vi "Handle Chart Settings.vi"(6 "Table Setting Name in":string, 7 "Write Ctl? (F:Read)":bool, 8 "error in (no error)":errorcluster, 9 "Table Ref":refnum<vi>, 11 "Save Restore Settings in":refnum<class "Save Restore Settings.lvclass">) -> (0 "error out":errorcluster, 1 "Sub Controls":T1[](array[typedef]), 3 "Save Restore Settings out":refnum<class "Save Restore Settings.lvclass">)   [LabVIEW 2016, in "Save Restore Settings.lvclass"]
uses:
  <userlib>/_MGI/Application Control/MGI Save Restore Settings/Save Restore Settings.lvclass
  <userlib>/_MGI/Application Control/MGI Save Restore Settings/Control Info.ctl
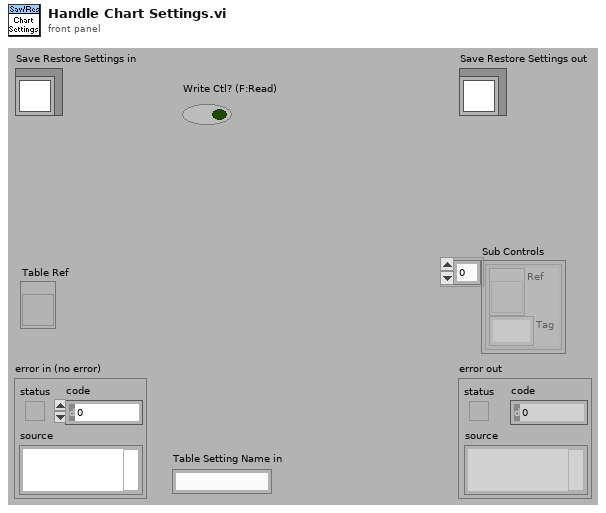
[diagram p1: front panel]
types:
  T1 = typedef "Save Restore Settings.lvclass/Control Info.ctl" = cluster{"Ref":refnum<vi>, "Tag":string}
  T2 = cluster{"XScaleIdx":u32, "YScaleIdx":u32, "Info":cluster{"Plot Color":u32, "Plot Interpolation":u8, "Point Style":u8, "Line Style":u8, "Fill/Pt. Color":u32, "Line Width":u8, "Bar Plot Style":u8, "Fill To":i16}}
  T3 = cluster{"Plot Color":u32, "Plot Interpolation":u8, "Point Style":u8, "Line Style":u8, "Fill/Pt. Color":u32, "Line Width":u8, "Bar Plot Style":u8, "Fill To":i16}
  T4 = cluster{"XScaleIdx":u32, "YScaleIdx":u32, "Info":cluster{"Plot Color":u32, "Plot Interpolation":u8, "Point Style":u8, "Line Style":u8, "Fill/Pt. Color":u32, "Line Width":u8, "Bar Plot Style":u8, "Fill To":i16}}[]
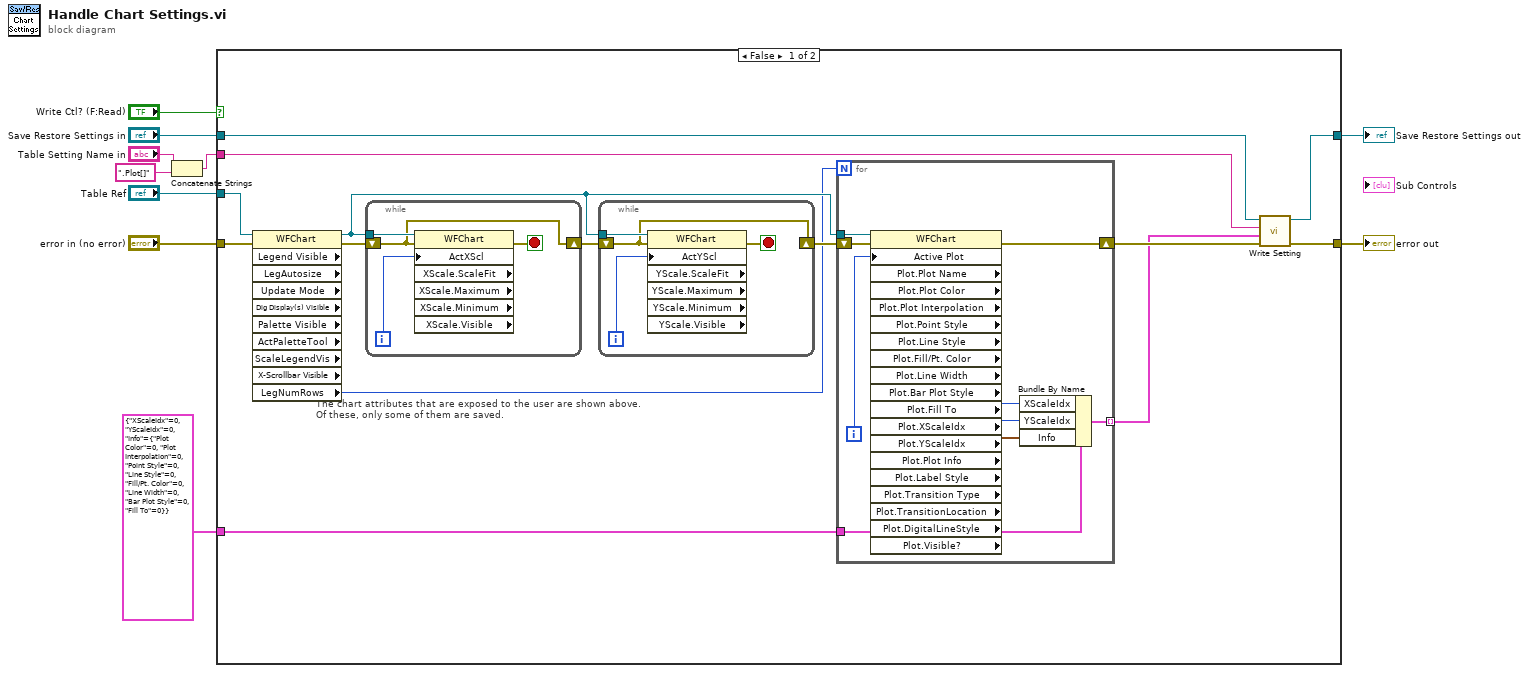
[diagram p0: block diagram]
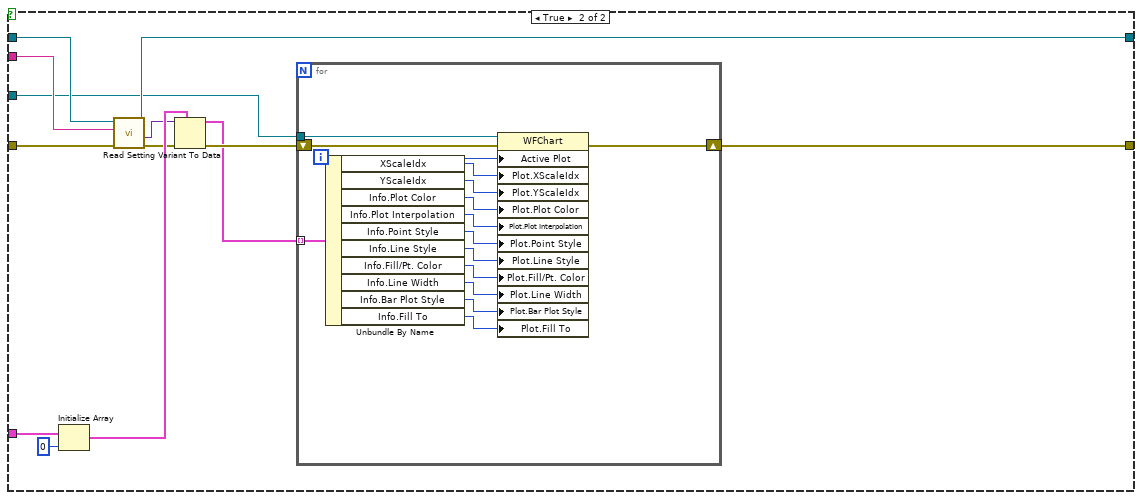
[diagram p2: hidden frame]
diagram:
  n1 = Concatenate Strings("Table Setting Name in", ".Plot[]" ("string")) -> (w2:string)
  n2 = case shown="False" "Write Ctl? (F:Read)" {
    tunnel: "Table Ref" -> [w24 w44]
    tunnel: "error in (no error)" -> [w23 w54]
    tunnel: "Save Restore Settings in" -> [w22 w48]
    tunnel: [w21 w47] -> w7
    tunnel: [w20 w43] -> w6
    tunnel: w2 -> [w12 w46]
    tunnel: T2 {"XScaleIdx"=0, "YScaleIdx"=0, "Info"={"Plot Color"=0, "Plot Interpolation"=0, "Point Style"=0, "Line Style"=0, "Fill/Pt. Color"=0, "Line Width"=0, "Bar Plot Style"=0, "Fill To"=0}} ("output cluster") -> [w11 w53]
    frame False {
      # "The chart attributes that are exposed to the user are shown above.\nOf these, only some of them are saved."
      n3 = property class="WFChart" props=["Legend Visible", "LegAutosize", "Update Mode", "Dig Display(s) Visible", "Palette Visible", "ActPaletteTool", "ScaleLegendVis", "X-Scrollbar Visible", "LegNumRows"](reference=w24, error in=w23) -> (reference out=w15:refnum<vi>, error out=w19:errorcluster, "LegNumRows"=w13:u32)  [unwired: 8 out]
      n4 = while {
        tunnel: w15 -> [w40]
        shift-right: [w39] -> w18
        shift-left: w19 -> [w39]
        i -> [w38]
        stop <- w41 stop-if-true
        n5 = property class="WFChart" props=["ActXScl", "XScale", "ScaleFit", "XScale", "Maximum", "XScale", "Minimum", "XScale", "Visible"](reference=w40, error in=w39, "ActXScl"=w38) -> (error out=w41:errorcluster)  [unwired: 5 out]
      }
      n6 = while {
        tunnel: w15 -> [w36]
        shift-right: [w35] -> w17
        shift-left: w18 -> [w35]
        i -> [w34]
        stop <- w37 stop-if-true
        n7 = property class="WFChart" props=["ActYScl", "YScale", "ScaleFit", "YScale", "Maximum", "YScale", "Minimum", "YScale", "Visible"](reference=w36, error in=w35, "ActYScl"=w34) -> (error out=w37:errorcluster)  [unwired: 5 out]
      }
      n8 = for {
        N: w13 -> [_]
        shift-right: [w30] -> w16
        shift-left: w17 -> [w33]
        tunnel: w15 -> [w32]
        tunnel: w11 -> [w26]
        tunnel: [w25] -> w14 mode=indexing
        i -> [w31]
        n9 = property class="WFChart" props=["Active Plot", "Plot", "Plot Name", "Plot", "Plot Color", "Plot", "Plot Interpolation", "Plot", "Point Style", "Plot", "Line Style", "Plot", "Fill/Pt. Color", "Plot", "Line Width", "Plot", "Bar Plot Style", "Plot", "Fill To", "Plot", "XScaleIdx", "Plot", "YScaleIdx", "Plot", "Plot Info", "Plot", "Label Style", "Plot", "Transition Type", "Plot", "TransitionLocation", "Plot", "DigitalLineStyle", "Plot", "Visible?"](reference=w32, error in=w33, "Active Plot"=w31) -> (error out=w30:errorcluster, "Plot.XScaleIdx"=w29:u32, "Plot.YScaleIdx"=w27:u32, "Plot.Plot Info"=w28:T3)  [unwired: 15 out]
        n10 = Bundle By Name(cluster=w26, "XScaleIdx"=w29, "YScaleIdx"=w27, "Info"=w28) -> (w25:T2)
      }
      n11 = call-dynamic "Write Setting.vi"("error in (no error)"=w16, "Tag Attribute"=w14, "Tag Name"=w12, "Save Restore Settings in"=w22) -> ("error out"=w20:errorcluster, "Save Restore Settings out"=w21:refnum<class "Save Restore Settings.lvclass">)  [unwired: 6 in]
    }
    frame True {
      n12 = Initialize Array(w53, 0 ("dimension size")) -> (w51:T4)
      n13 = call-dynamic "Read Setting.vi"("error in (no error)"=w54, "Tag Name"=w46, "Save Restore Settings in"=w48) -> ("error out"=w50:errorcluster, "Tag Attribute"=w49:variant, "Save Restore Settings out"=w47:refnum<class "Save Restore Settings.lvclass">)  [unwired: 6 in]
      n14 = Variant To Data(error in=w50, type=w51, Variant=w49) -> (data=w42:T4, error out=w45:errorcluster)
      n15 = for {
        shift-right: [w68] -> w43
        shift-left: w45 -> [w69]
        tunnel: w44 -> [w67]
        tunnel: w42 -> [w65] mode=indexing
        i -> [w66]
        n16 = Unbundle By Name(w65) -> ("XScaleIdx"=w64:u32, "YScaleIdx"=w63:u32, "Info.Plot Color"=w61:u32, "Info.Plot Interpolation"=w62:u8, "Info.Point Style"=w60:u8, "Info.Line Style"=w59:u8, "Info.Fill/Pt. Color"=w58:u32, "Info.Line Width"=w57:u8, "Info.Bar Plot Style"=w56:u8, "Info.Fill To"=w55:i16)
        n17 = property class="WFChart"(reference=w67, error in=w69, "Active Plot"=w66, "Plot.XScaleIdx"=w64, "Plot.YScaleIdx"=w63, "Plot.Plot Color"=w61, "Plot.Plot Interpolation"=w62, "Plot.Point Style"=w60, "Plot.Line Style"=w59, "Plot.Fill/Pt. Color"=w58, "Plot.Line Width"=w57, "Plot.Bar Plot Style"=w56, "Plot.Fill To"=w55) -> (error out=w68:errorcluster)  [unwired: 1 out]
      }
    }
  }
  "error out" <- w6
  "Save Restore Settings out" <- w7
